vi "reconstructPath.vi"(8 "error in (no error)":errorcluster, 10 "path in":T1[](array[typedef]), 11 "Waypoint in":refnum<class "Waypoint.lvclass">) -> (0 "error out":errorcluster, 2 "path out":T1[](array[typedef]), 3 "Waypoint out":refnum<class "Waypoint.lvclass">)   [LabVIEW 2009, in "Waypoint.lvclass"]
uses:
  Waypoint.lvclass
  TreeNode/TreeNode.lvclass
  point.ctl
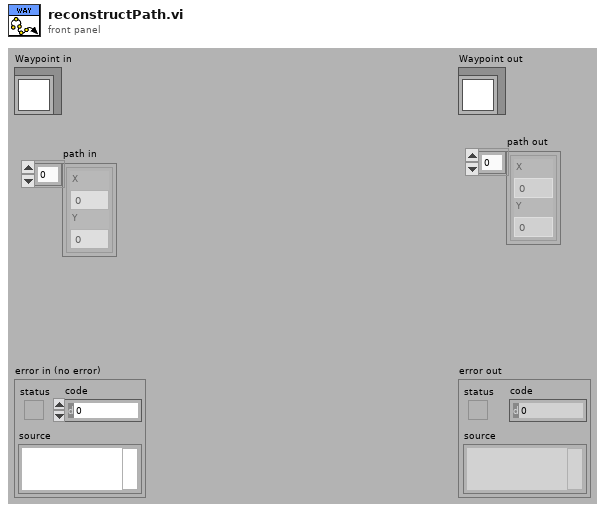
[diagram p1: front panel]
types:
  T1 = typedef "Waypoint.lvclass/point.ctl" = cluster{"X":dbl, "Y":dbl}
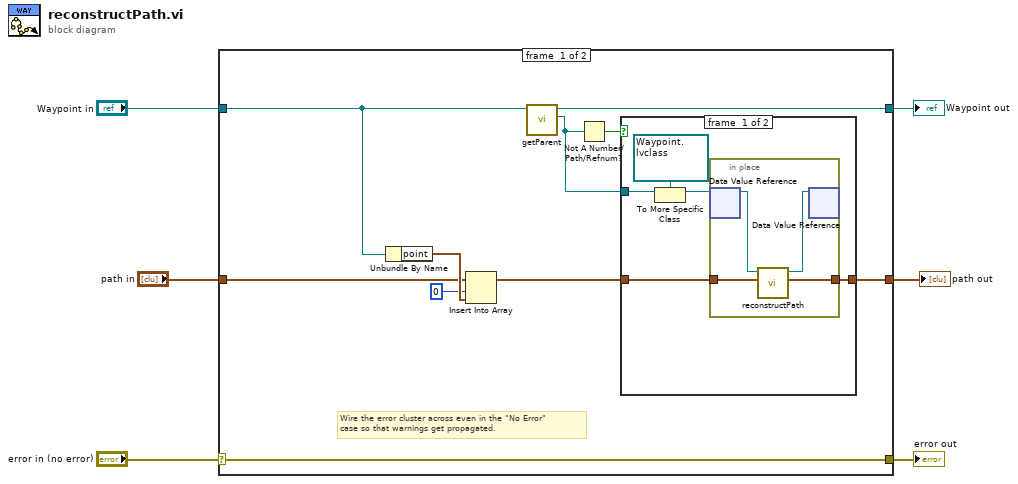
[diagram p0: block diagram]
diagram:
  n1 = case shown="No Error" "error in (no error)" {
    selector: "error in (no error)" -> [w16 w28]
    tunnel: [w16 w28] -> w5
    tunnel: [w9 w27] -> w3
    tunnel: "Waypoint in" -> [w13 w27]
    tunnel: "path in" -> [w14 _]
    tunnel: [w10 _] -> w1
    frame #0 {
      # "Wire the error cluster across even in the \"No Error\"\ncase so that warnings get propagated."
      n2 = Unbundle By Name(w13) -> ("point"=w15:T1)
      n3 = Insert Into Array(array=w14, index=0, new element=w15) -> (w11:T1[])
      n4 = call "getParent.vi"("TreeNode in"=w13) -> ("Parent"=w8:refnum<data-value>, "TreeNode out"=w9:refnum<class "Waypoint.lvclass">)  [unwired: 8 in, 1 out]
      n5 = Not A Number/Path/Refnum?(number/path/refnum=w8) -> (NaN/Path/Refnum?=w12:bool)
      n6 = case shown="False" w12 {
        tunnel: w11 -> [w19 w26]
        tunnel: [w17 w26] -> w10
        tunnel: w8 -> [w21 _]
        frame #0 {
          n7 = To More Specific Class(target class=refnum<data-value> refnum ("data value reference"), reference=w21) -> (specific class reference=w18:refnum<data-value>)  [unwired: 1 in, 1 out]
          n8 = in-place {
            in-place-border: w19 -> [w25]
            in-place-border: [w24] -> w17
            n9 = in-place-dvr #1(w18) -> (w23:refnum<class "Waypoint.lvclass">)  [unwired: 1 out]
            n10 = call "reconstructPath.vi"("path in"=w25, "Waypoint in"=w23) -> ("path out"=w24:T1[], "Waypoint out"=w22:refnum<class "Waypoint.lvclass">)  [unwired: 7 in, 1 out]
            n11 = in-place-dvr #1(w22) -> ()  [unwired: 2 out]
          }
        }
        frame #1 {
        }
      }
    }
    frame #1 {
    }
  }
  "error out" <- w5
  "Waypoint out" <- w3
  "path out" <- w1
